vi "SP Convert Delta to Upper - Lower.vi"(4 "Limits":T1[](array[typedef]) {"Parameter"."Stimulus Port" min=1 step=1; "Parameter"."Response Port" min=1 step=1}) -> (1 "Converted Limits":T1[](array[typedef]) {"Parameter"."Stimulus Port" min=1 step=1; "Parameter"."Response Port" min=1 step=1})   [LabVIEW 2011]
uses:
  TypeDefs/SP Limit.ctl
  TypeDefs/SP Parameter.ctl
  TypeDefs/SP Format.ctl
  TypeDefs/SP Limit Type.ctl
  TypeDefs/SP Limit Point.ctl
  Test Referential Limit.ctl
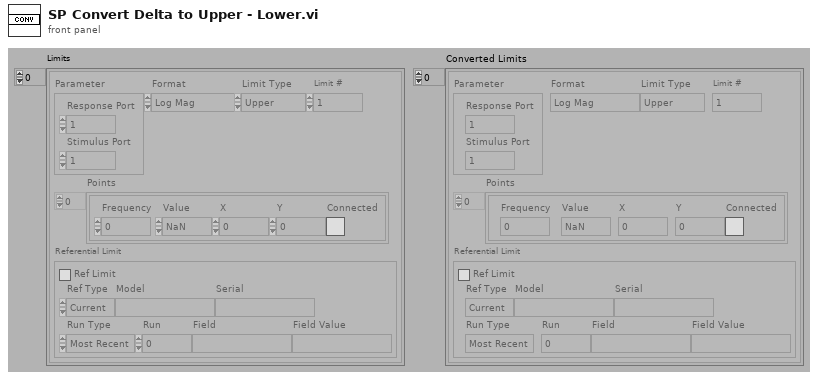
[diagram p1: front panel]
types:
  T1 = typedef "SP Limit.ctl" = cluster{"Parameter":T2, "Format":T3, "Limit Type":T4, "Points":T5[], "Referential Limit":T6, "Limit #":i8}
  T2 = typedef "SP Parameter.ctl" = cluster{"Stimulus Port":i8, "Response Port":i8}
  T3 = typedef "SP Format.ctl" = enum16{"Log Mag", "Lin Mag", "SWR", "Phase", "Expanded Phase", "Delay", "Insertion Loss", "Isolation", "Return Loss"}
  T4 = typedef "SP Limit Type.ctl" = enum16{"Upper", "Lower", "Delta", "Filter", "Referential"}
  T5 = typedef "SP Limit Point.ctl" = cluster{"Frequency":dbl, "Value":dbl, "X":dbl, "Y":dbl, "Connected":bool}
  T6 = typedef "Test Referential Limit.ctl" = cluster{"Ref Limit":bool, "Ref Type":enum16{"Current", "Specify"}, "Model":string, "Serial":string, "Run Type":enum16{"Most Recent", "Run #", "Match Field"}, "Run":i32, "Field":string, "Field Value":string}
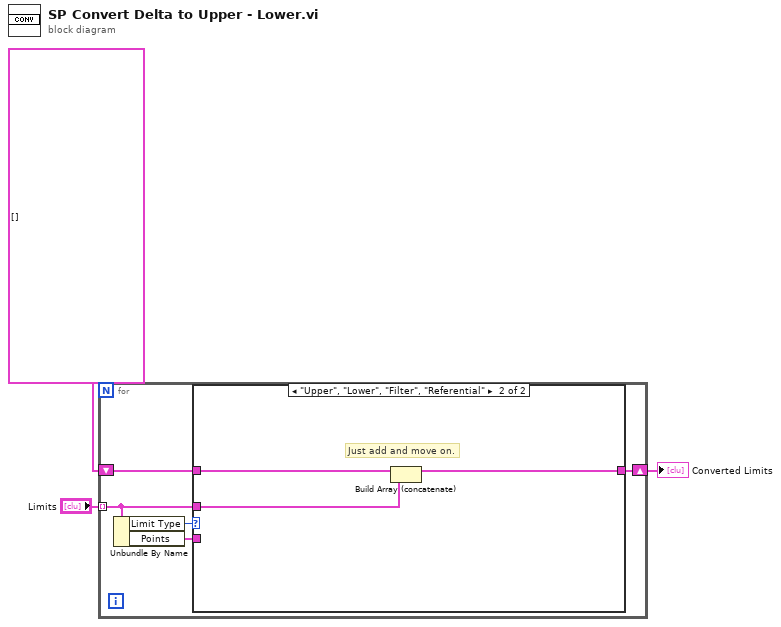
[diagram p0: block diagram]
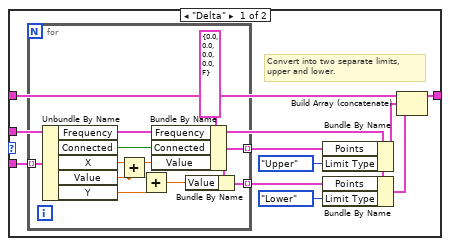
[diagram p2: hidden frame]
diagram:
  n1 = for {
    tunnel: "Limits" -> [w6] mode=indexing
    shift-right: [w5] -> w1
    shift-left: T1[] [] ("Limits") -> [w4]
    n2 = Unbundle By Name(w6) -> ("Limit Type"=w7:T4, "Points"=w8:T5[])
    n3 = case shown="\"Upper\", \"Lower\", \"Filter\", \"Referential\"" w7 {
      tunnel: w8 -> [w18 _]
      tunnel: w6 -> [w15 w32]
      tunnel: [w10 w30] -> w5
      tunnel: w4 -> [w9 w31]
      frame "Delta" {
        # "Convert into two separate limits,\nupper and lower."
        n4 = for {
          tunnel: w18 -> [w29] mode=indexing
          tunnel: [w20] -> w17 mode=indexing
          tunnel: [w19] -> w16 mode=indexing
          n5 = Unbundle By Name(w29) -> ("Frequency"=w28:dbl, "Connected"=w26:bool, "X"=w25:dbl, "Value"=w22:dbl, "Y"=w23:dbl)
          n6 = Add(x=w25, y=w22) -> (x+y=w24:dbl)
          n7 = Add(x=w22, y=w23) -> (x+y=w21:dbl)
          n8 = Bundle By Name(cluster=T5 {"Frequency"=0.0, "Value"=0.0, "X"=0.0, "Y"=0.0, "Connected"=FALSE} ("Point"), "Frequency"=w28, "Connected"=w26, "Value"=w24) -> (w20:T5)
          n9 = Bundle By Name(cluster=w20, "Value"=w21) -> (w19:T5)
        }
        n10 = Bundle By Name(cluster=w15, "Points"=w17, "Limit Type"=enum16{"Upper", "Lower", "Delta"}."Upper") -> (w12:T1)
        n11 = Bundle By Name(cluster=w15, "Points"=w16, "Limit Type"=enum16{"Upper", "Lower", "Delta"}."Lower") -> (w11:T1)
        n12 = Build Array (concatenate)(w9, w12, w11) -> (w10:T1[])
      }
      frame "Upper", "Lower", "Filter", "Referential" {
        # "Just add and move on."
        n13 = Build Array (concatenate)(w31, w32) -> (w30:T1[])
      }
    }
  }
  "Converted Limits" <- w1
